vi "myRIO_BRig_RT_dataExp_laser1_Tshutter.vi"() -> (2 "output_laser1_Tshutter":i32)   [LabVIEW 2014]
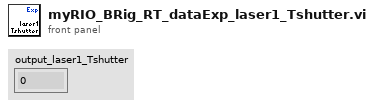
[diagram p1: front panel]
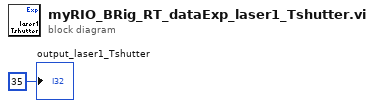
[diagram p0: block diagram]
diagram:
  "output_laser1_Tshutter" <- 35 ("output_iBlock")
